vi "Create List.vi"(9 "Indicator":bool, 10 "Label.Text":string, 11 "VI in":refnum<vi>) -> (2 "format string":string, 3 "String":string)   [LabVIEW 2019]
uses:
  <vilib>/Utility/Data Type/NI_Data Type.lvlib
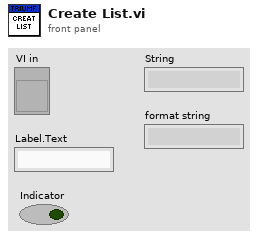
[diagram p1: front panel]
types:
  T1 = typedef "NI_Data Type.lvlib/Data Type.ctl" = enum8{"Invalid Type", "Void", "I8", "I16", "I32", "I64", "U8", "U16", "U32", "U64", "Single Float", "Double Float", "Extended Float", "Single Complex", "Double Complex", "Extended Complex", "Enum U8", "Enum U16", "Enum U32", "Enum U64", "Single Float With Unit", "Double Float With Unit", "Extended Float With Unit", "Single Complex with Unit", "Double Complex with Unit", "Extended Complex with Unit", "Boolean", "String", "Path", "Picture", "Tag", "Array", "Cluster", "Variant", "LV Variant", "Waveform", "Timestamp", "Digital Waveform", "Digital Data", "ExpressData", "Refnum", "External Data", "VI", "Poly VI", "LabVIEW Class Instance", "Fixed Point", "Set Collection", "Map Collection"}
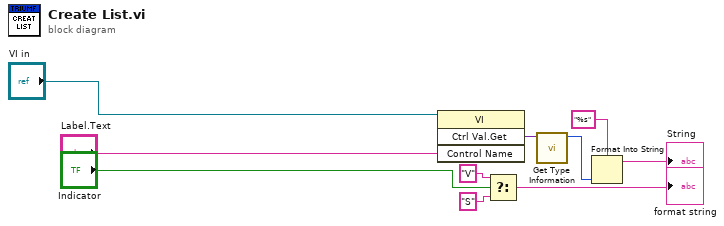
[diagram p0: block diagram]
diagram:
  n1 = invoke class="VI" method="Ctrl Val.Get"(reference="VI in", "Control Name"="Label.Text") -> ("Get Control Value Variant"=w4:variant)  [unwired: 2 in, 3 out]
  n2 = Select(t="V" ("format string"), s="Indicator", f="S" ("format string")) -> (s? t:f=→"format string":string)
  n3 = call <vilib>:"Get Type Information.vi"("variant"=w4) -> ("type"=w2:T1)  [unwired: 6 in, 4 out]
  n4 = Format Into String(format string="%s", w2) -> (resulting string=→"String":string)  [unwired: 2 in, 1 out]
